vi "helloworld.vi"() -> ()   [LabVIEW 2016]
panel:
  in  "stop":bool
  in  "Do work":bool
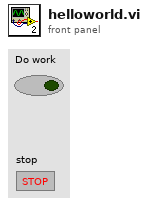
[diagram p1: front panel]
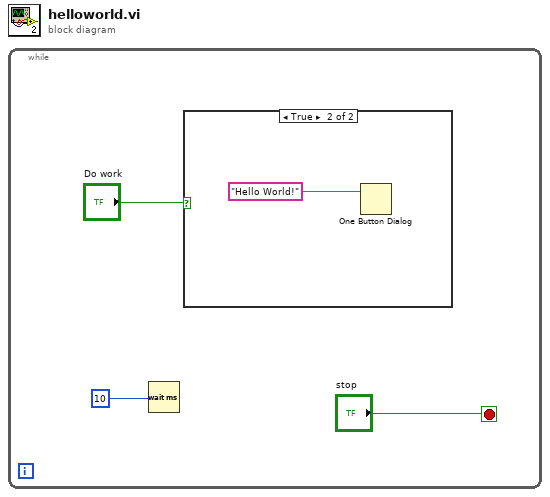
[diagram p0: block diagram]
diagram:
  n1 = while {
    stop <- "stop" stop-if-true
    n2 = Wait (ms)(milliseconds to wait=10) -> ()  [unwired: 1 out]
    n3 = case shown="True" "Do work" {
      frame False {
      }
      frame True {
        n4 = One Button Dialog(message="Hello World!") -> ()  [unwired: 1 in, 1 out]
      }
    }
  }
